vi "TEST_ASIC_COMPLETE_(ALL)_NEW.vi"() -> ()   [LabVIEW 2012]
uses:
  <vilib>/Utility/NIReport.llb/HTML/NI_HTML.lvclass
  <vilib>/Utility/NIReport.llb/NI_report.lvclass
panel:
  in  "Baseline":bool
  in  "Majority Test":bool
  in  "SumNAdder\n      Test":bool=TRUE
  in  "Sum Test":bool
  in  "Instrument VISA in":T1={"AWG VISA"="AgilentGenerator1", "Oscilloscope  VISA "="AgilentOsciloscope", "Integration Board IP"="172.16.17.47", "connection ID"=refnum, "report out"=refnum, "report file path"=path "C:/Users/omartinez/Desktop/L0nL1_Results"}
  out "Instrument VISA out":T1={"AWG VISA"="AgilentGenerator1", "Oscilloscope  VISA "="AgilentOsciloscope", "Integration Board IP"="172.16.7.43", "connection ID"=refnum, "report out"=refnum, "report file path"=path "C:/Users/omartinez/Desktop/L0nL1_Results"}
  out "error out":errorcluster
  in  "error in":errorcluster
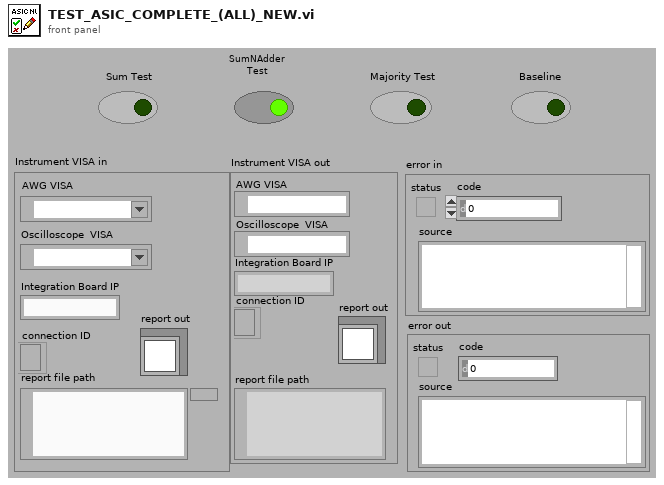
[diagram p1: front panel]
types:
  T1 = cluster{"AWG VISA":refnum<visa-resource-name>, "Oscilloscope  VISA ":refnum<visa-resource-name>, "Integration Board IP":string, "connection ID":refnum<k5>, "report out":refnum<class "NI_report.lvclass">, "report file path":path}
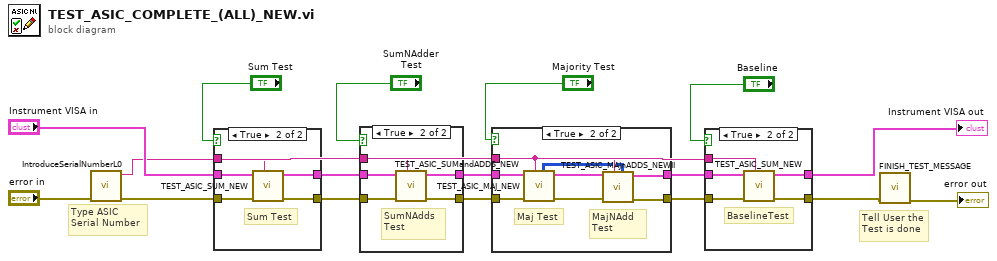
[diagram p0: block diagram]
diagram:
  # "Tell User the\nTest is done"
  # "Type ASIC\nSerial Number"
  n1 = call "IntroduceSerialNumberL0.vi"("error in"="error in") -> ("error out"=w3:errorcluster, "Serial Number"=w1:string)  [unwired: 9 in]
  n2 = case shown="True" "Sum Test" {
    tunnel: [w19 w21] -> w17
    tunnel: [w18 w24] -> w15
    tunnel: "Instrument VISA in" -> [w19 w22]
    tunnel: w3 -> [w18 w23]
    tunnel: w1 -> [_ w20]
    frame False {
    }
    frame True {
      # "Sum Test"
      n3 = call "TEST_ASIC_SUM_NEW.vi"("Serial Number"=w20, "error in (no error)"=w23, "Instrument VISA in"=w22) -> ("error out"=w24:errorcluster, "Instrument VISA out 2"=w21:T1)  [unwired: 7 in]
    }
  }
  n4 = case shown="True" "SumNAdder\n      Test" {
    tunnel: w17 -> [w26 w29]
    tunnel: [w26 w28] -> w16
    tunnel: w15 -> [w25 w31]
    tunnel: [w25 w30] -> w14
    tunnel: w1 -> [_ w27]
    frame False {
    }
    frame True {
      # "SumNAdds\nTest"
      n5 = call "TEST_ASIC_SUMandADDS_NEW.vi"("Serial Number"=w27, "error in (no error)"=w31, "Instrument VISA in"=w29) -> ("error out"=w30:errorcluster, "Instrument VISA out"=w28:T1)  [unwired: 7 in]
    }
  }
  n6 = case shown="True" "Majority Test" {
    tunnel: w16 -> [w33 w40]
    tunnel: [w33 w36] -> w6
    tunnel: w14 -> [w32 w41]
    tunnel: [w32 w39] -> w7
    tunnel: w1 -> [_ w35]
    frame False {
    }
    frame True {
      # "MajNAdd\nTest"
      # "Maj Test"
      n7 = call "TEST_ASIC_MAJ_NEW.vi"("Serial Number"=w35, "error in"=w41, "Instrument VISA in"=w40) -> ("error out"=w38:errorcluster, "Instrument VISA out"=w37:T1, "ThresholdOut"=w34:i32[][])  [unwired: 6 in]
      n8 = call "TEST_ASIC_MAJnADDS_NEWII.vi"("threshold"=w34, "Serial Number"=w35, "error in"=w38, "Instrument VISA in"=w37) -> ("error out"=w39:errorcluster, "Instrument VISA out"=w36:T1)  [unwired: 6 in]
    }
  }
  n9 = case shown="True" "Baseline" {
    tunnel: [w43 w45] -> w4
    tunnel: [w42 w48] -> w5
    tunnel: w6 -> [w43 w46]
    tunnel: w7 -> [w42 w47]
    tunnel: w1 -> [_ w44]
    frame False {
    }
    frame True {
      # "BaselineTest"
      n10 = call "TEST_ASIC_SUM_NEW.vi"("Serial Number"=w44, "error in (no error)"=w47, "Instrument VISA in"=w46) -> ("error out"=w48:errorcluster, "Instrument VISA out 2"=w45:T1)  [unwired: 7 in]
    }
  }
  "Instrument VISA out" <- w4
  n11 = call "FINISH_TEST_MESSAGE.vi"("error in"=w5) -> ("error out"=→"error out":errorcluster)  [unwired: 10 in]
